vi "Get Active Observer.vi"(8 "error in (no error)":errorcluster, 11 "Vessel in":refnum<class "Vessel.lvclass">) -> (0 "error out":errorcluster, 2 "Active Observer":refnum<class "Observer.lvclass">, 3 "Vessel out":refnum<class "Vessel.lvclass">)   [LabVIEW 2014, in "Vessel.lvclass"]
uses:
  Vessel.lvclass
  Observer/Observer.lvclass
  Vessel.lvclass/Vessel.ctl
  Supervisor/Supervisor.lvclass
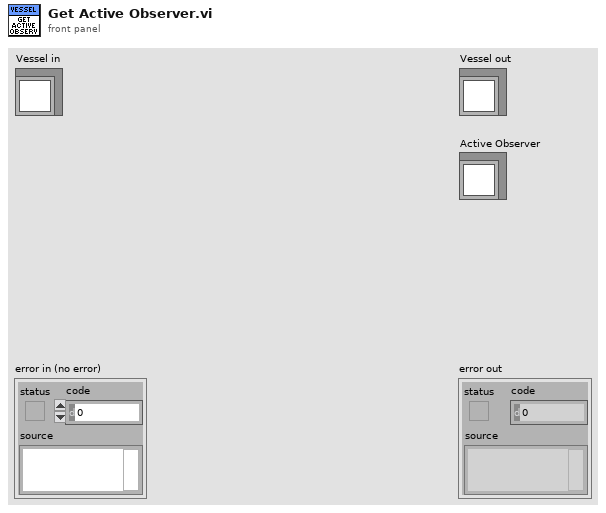
[diagram p1: front panel]
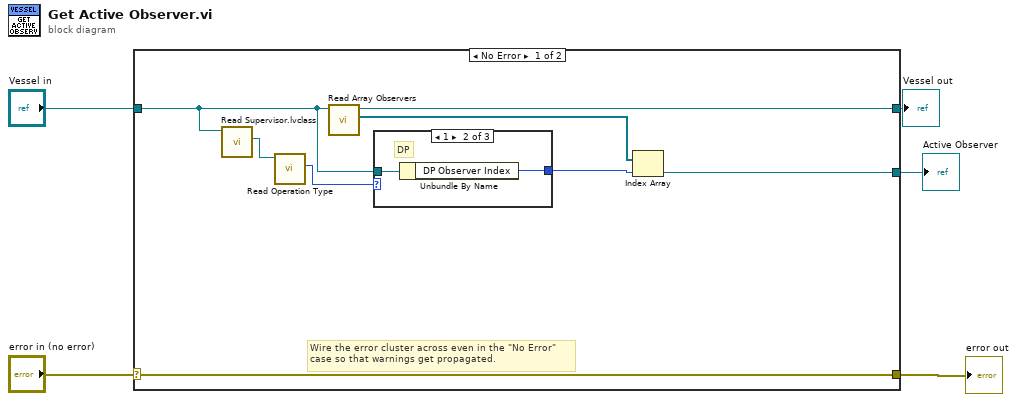
[diagram p0: block diagram]
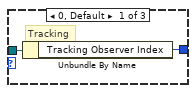
[diagram p2: hidden frame]
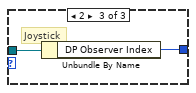
[diagram p3: hidden frame]
diagram:
  n1 = case shown="No Error" "error in (no error)" {
    selector: "error in (no error)" -> [w13 w21]
    tunnel: [w13 w21] -> w4
    tunnel: [w9 w20] -> w2
    tunnel: "Vessel in" -> [w10 w20]
    tunnel: [w7 _] -> w1
    frame No Error {
      # "Wire the error cluster across even in the \"No Error\"\ncase so that warnings get propagated."
      n2 = call "Read Supervisor.lvclass.vi"("Vessel in"=w10) -> ("Supervisor.lvclass"=w12:refnum<class "Supervisor.lvclass">)  [unwired: 8 in, 2 out]
      n3 = call-dynamic "Read Operation Type.vi"("Supervisor in"=w12) -> ("Operation Type"=w11:u16)  [unwired: 8 in, 2 out]
      n4 = call-dynamic "Read Array Observers.vi"("Vessel in"=w10) -> ("Array Observers"=w8:refnum<class "Observer.lvclass">[], "Vessel out"=w9:refnum<class "Vessel.lvclass">)  [unwired: 8 in, 1 out]
      n5 = case shown="1" w11 {
        tunnel: w10 -> [w15 w17 w19]
        tunnel: [w14 w16 w18] -> w6
        frame 0, Default {
          # "Tracking"
          n6 = Unbundle By Name(w15) -> ("Tracking Observer Index"=w14:i32)
        }
        frame 1 {
          # "DP"
          n7 = Unbundle By Name(w17) -> ("DP Observer Index"=w16:i32)
        }
        frame 2 {
          # "Joystick"
          n8 = Unbundle By Name(w19) -> ("DP Observer Index"=w18:i32)
        }
      }
      n9 = Index Array(array=w8, index=w6) -> (element=w7:refnum<class "Observer.lvclass">)
    }
    frame Error {
    }
  }
  "error out" <- w4
  "Vessel out" <- w2
  "Active Observer" <- w1
